vi "Configure Interlock Threshold Level.vi"(8 "error in (no error)":errorcluster, 10 "Threshold Voltage Level (42 V)":dbl=42.0, 11 "VISA resource name":refnum<visa-resource-name>) -> (0 "error out":errorcluster, 3 "VISA resource name out":refnum<visa-resource-name>)   [LabVIEW 2026, in "Agilent B2900 Series.lvlib"]
doc: "Configures the interlock threshold voltage level of all channels. The setting is stored in the non-volatile memory.\n\n<b>Note(s)</b>\nThis VI is only applicable for B2901CL, B2901C, B2902C, B2910CL, B2911C, B2912C, B2961C, B2962C models."
uses:
  Agilent B2900 Series.lvlib
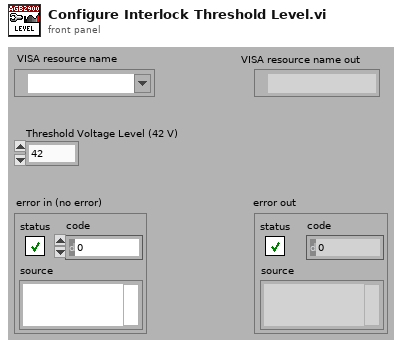
[diagram p1: front panel]
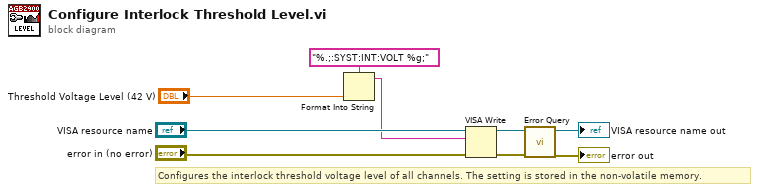
[diagram p0: block diagram]
diagram:
  # "Configures the interlock threshold voltage level of all channels. The setting is stored in the non-volatile memory."
  n1 = Format Into String(format string="%.;:SYST:INT:VOLT %g;", "Threshold Voltage Level (42 V)") -> (resulting string=w1:string)  [unwired: 2 in, 1 out]
  n2 = VISA Write(VISA resource name="VISA resource name", write buffer=w1, error in (no error)="error in (no error)") -> (VISA resource name out=w7:refnum<visa-resource-name>, error out=w6:errorcluster)  [unwired: 1 out]
  n3 = call "Error Query.vi"("error in (no error)"=w6, "VISA resource name"=w7) -> ("error out"=→"error out":errorcluster, "VISA resource name out"=→"VISA resource name out":refnum<visa-resource-name>)  [unwired: 6 in, 2 out]
